vi "Read Engine Cluster.vi"(8 "error in (no error)":errorcluster, 11 "Abstract Engine in":refnum<class "Abstract Engine.lvclass">) -> (0 "error out":errorcluster, 2 "Engine Cluster":T1, 3 "Abstract Engine out":refnum<class "Abstract Engine.lvclass">)   [LabVIEW 2025, in "Abstract Engine.lvlib" / "Abstract Engine.lvclass"]
uses:
  Abstract Engine.lvclass
  Engine Cluster.ctl
  Abstract Instrument/Channel.ctl
  Abstract Engine.lvclass/Abstract Engine.ctl
  Abstract Instrument/Abstract Instrument.lvclass
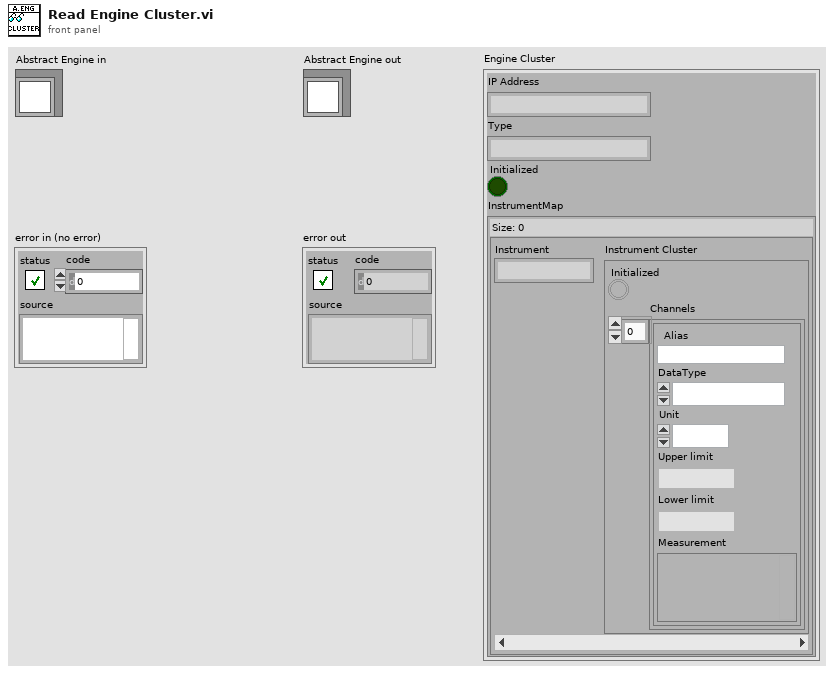
[diagram p1: front panel]
types:
  T1 = typedef "Abstract Engine.lvlib/Abstract Engine.lvclass/Engine Cluster.ctl" = cluster{"IP Address":string, "Type":string, "Initialized":bool, "InstrumentMap":map{string, cluster{"Initialized":bool, "Channels":T2[]}}}
  T2 = typedef "Abstract Engine.lvlib/Abstract Instrument.lvclass/Channel.ctl" = cluster{"Alias":string, "DataType":enum16{"Anaolg Input", "Waveform"}, "Unit":enum16{"---", "V", "A", "Ohm", "Hz", "uF", "degC", "deg"}, "Upper limit":dbl, "Lower limit":dbl, "Measurement":variant}
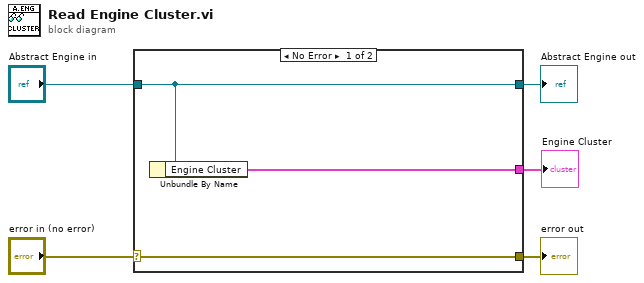
[diagram p0: block diagram]
diagram:
  n1 = case shown="No Error" "error in (no error)" {
    selector: "error in (no error)" -> [w8 w9]
    tunnel: [w8 w9] -> w4
    tunnel: [w7 w10] -> w2
    tunnel: "Abstract Engine in" -> [w7 w10]
    tunnel: [w6 _] -> w1
    frame No Error {
      n2 = Unbundle By Name(w7) -> ("Engine Cluster"=w6:T1)
    }
    frame Error {
    }
  }
  "error out" <- w4
  "Abstract Engine out" <- w2
  "Engine Cluster" <- w1
